vi "sub_转换成偶数数组.vi"(1 "输入数组":i32[](array[numeric])) -> (0 "输出数组":i32[](array[numeric]))   [LabVIEW 2015]
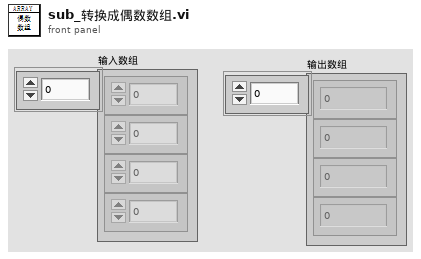
[diagram p1: front panel]
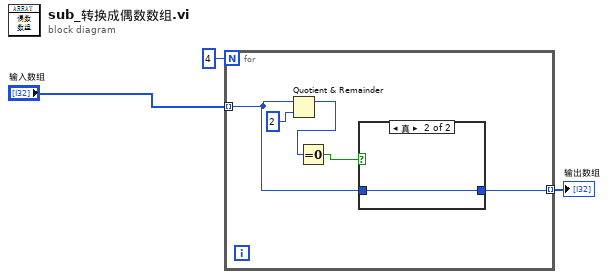
[diagram p0: block diagram]
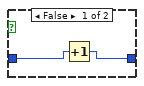
[diagram p2: hidden frame]
diagram:
  n1 = for {
    N: 4 -> [_]
    tunnel: "输入数组" -> [w5] mode=indexing
    tunnel: [w6] -> w1 mode=indexing
    n2 = Quotient & Remainder(x=w5, y=2) -> (x-y*floor(x/y)=w4:i32)  [unwired: 1 out]
    n3 = Equal To 0?(x=w4) -> (x = 0?=w7:bool)
    n4 = case shown="真" w7 {
      tunnel: [w9 w11] -> w6
      tunnel: w5 -> [w10 w11]
      frame False {
        n5 = Increment(x=w10) -> (x+1=w9:i32)
      }
      frame True {
      }
    }
  }
  "输出数组" <- w1
